vi "LVClass_WavefrontCorrectorSet get ActionName.vi"(0 "WavefrontCorrectorSet in":refnum<class "WavefrontCorrectorSet.lvclass">, 5 "index":i32, 11 "error in (no error)":errorcluster) -> (4 "WavefrontCorrectorSet out":refnum<class "WavefrontCorrectorSet.lvclass">, 6 "Action Name":string, 15 "error out":errorcluster)   [LabVIEW 2020, in "WavefrontCorrectorSet.lvclass"]
doc: "WavefrontCorrector features name getter given its position in the parameters\nlist.\n\n--------------------------------------------------------------------------------\n\n<B>wavefrontcorrector_setIn </B> : WavefrontCorrectorSet object.\n<B>wavefrontcorrector_setOut </B> : WavefrontCorrectorSet object.\n<B>index </B> : Feature index.\n<B>feature_name </B> : Feature name.\n<B>ErrorIn </B> : Error\n<B>ErrorOut </B> : Error\n\n--------------------------------------------------------------------------------"
uses:
  WavefrontCorrectorSet.lvclass
  WavefrontCorrectorSet.lvclass/WavefrontCorrectorSet.ctl
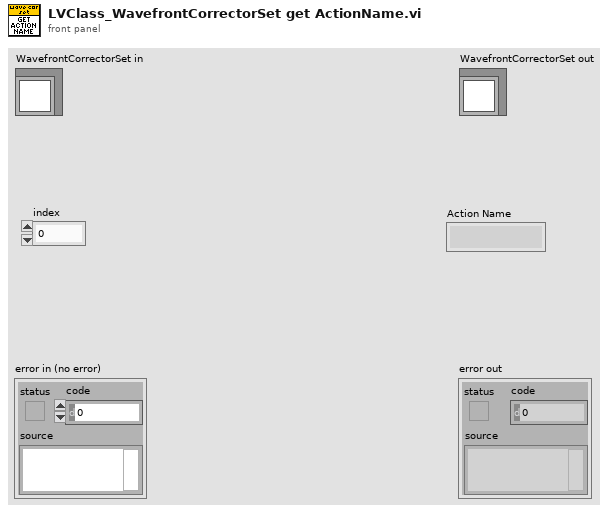
[diagram p1: front panel]
types:
  T1 = typedef "ClassID.ctl" = i64
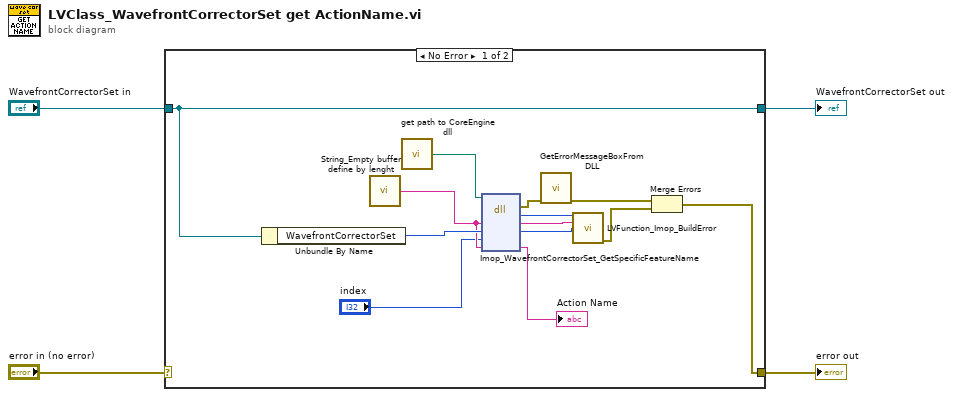
[diagram p0: block diagram]
diagram:
  n1 = case shown="No Error" "error in (no error)" {
    selector: "error in (no error)" -> [_ w19]
    tunnel: [w10 w19] -> w4
    tunnel: [w9 w18] -> w3
    tunnel: "WavefrontCorrectorSet in" -> [w9 w18]
    frame No Error {
      n2 = Unbundle By Name(w9) -> ("WavefrontCorrectorSet"=w11:T1)
      n3 = call "String_Empty buffer define by lenght.vi"() -> ("Empty buffer"=w8:string)  [unwired: 1 in]
      n4 = call "get path to CoreEngine dll.vi"() -> ("path to wavekit library"=w15:path)  [unwired: 14 in, 1 out]
      n5 = dll-call lib="D:/soft/HASO_v3/SVN_trunk/ImOpCoreEngine4_LV2011/DLLs/c_interface_vc100.dll" fn="Imop_WavefrontCorrectorSet_GetSpecificFeatureName"(path in=w15, "message"=w8, "WavefrontCorrectionSet"=w11, "index"="index", "Action Name"=w8) -> (error out=w14:errorcluster, "return type"=w17:i32, "message"=w16:string, "WavefrontCorrectionSet"=w5:i64, "Action Name"=→"Action Name":string)  [unwired: 3 in, 1 out]
      n6 = call "GetErrorMessageBoxFromDLL.vi"("error IN"=w14) -> ("error OUT"=w13:errorcluster)  [unwired: 10 in]
      n7 = call "LVFunction_Imop_BuildError.vi"("code"=w17, "String to Prepend to source (\"\")"=w16, "Adresse"=w5) -> ("error out"=w12:errorcluster)  [unwired: 12 in]
      n8 = Merge Errors(w13, w12) -> (w10:errorcluster)
    }
    frame Error {
    }
  }
  "error out" <- w4
  "WavefrontCorrectorSet out" <- w3
